vi "Get Slice Color.vi"(7 "Opacity":sgl, 9 "Normal Array":cluster{"X":sgl, "Y":sgl, "Z":sgl}[](array[cluster]), 11 "Color Pair Array":cluster{"Color":u32, "String":string}[](array[cluster])) -> (1 "Color Array":cluster{"R":sgl, "G":sgl, "B":sgl, "A":sgl}[](array[cluster]), 3 "Color Binding Mode":T1(ring))   [LabVIEW 2017, in "3D Pie.lvclass"]
uses:
  <vilib>/Math Plots/3D Math Plots/3D Pie/3D Pie/3D Pie.lvclass
  <vilib>/picture/3D Picture Control/NI_3D Picture Control.lvlib
  <vilib>/Math Plots/3D Math Plots/3D Plot/3D Plot/3D Plot.lvclass
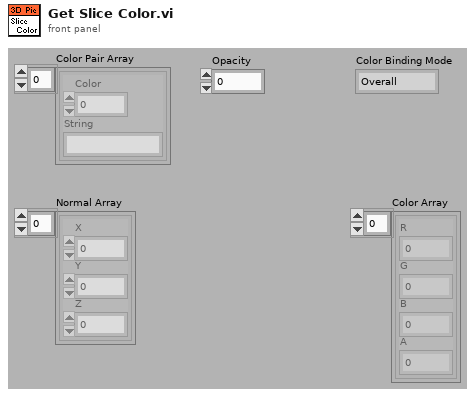
[diagram p1: front panel]
types:
  T1 = enum16{"Overall", "Per Primitive", "Per Vertex", "Binding Off"}
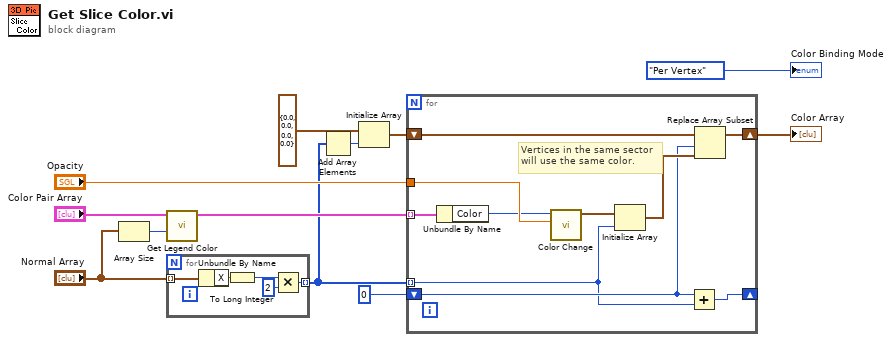
[diagram p0: block diagram]
diagram:
  n1 = Array Size(array="Normal Array") -> (size(s)=w6:i32)
  n2 = call <vilib>:"Get Legend Color.vi"("Pair Array Length"=w6, "Color Pair Array In"="Color Pair Array") -> ("Color Pair Array Out"=w8:cluster{"Color":u32, "String":string}[])  [unwired: 9 out]
  n3 = for {
    tunnel: "Normal Array" -> [w16] mode=indexing
    tunnel: [w13] -> w2 mode=indexing
    n4 = Unbundle By Name(w16) -> ("X"=w17:sgl)
    n5 = To Long Integer(number=w17) -> (32bit integer=w14:i32)
    n6 = Multiply(x=w14, y=2) -> (x*y=w13:i32)
  }
  n7 = Add Array Elements(numeric array=w2) -> (sum=w1:i32)
  n8 = Initialize Array(cluster{"R":sgl, "G":sgl, "B":sgl, "A":sgl} {"R"=0.0, "G"=0.0, "B"=0.0, "A"=0.0} ("RGBA"), w1) -> (w5:cluster{"R":sgl, "G":sgl, "B":sgl, "A":sgl}[])
  n9 = for {
    shift-right: [w26] -> w11
    shift-left: w5 -> [w27]
    tunnel: "Opacity" -> [w24]
    tunnel: w8 -> [w23] mode=indexing
    shift-right: [w19] -> _
    shift-left: 0 -> [w20]
    tunnel: w2 -> [w18] mode=indexing
    # "Vertices in the same sector\nwill use the same color."
    n10 = Unbundle By Name(w23) -> ("Color"=w22:u32)
    n11 = call <vilib>:"Color Change.vi"("Alpha"=w24, "Color"=w22) -> ("RGBA"=w25:cluster{"R":sgl, "G":sgl, "B":sgl, "A":sgl})  [unwired: 9 out]
    n12 = Initialize Array(w25, w18) -> (w21:cluster{"R":sgl, "G":sgl, "B":sgl, "A":sgl}[])
    n13 = Add(x=w20, y=w18) -> (x+y=w19:i32)
    n14 = Replace Array Subset(array=w27, new element=w21, index=w20) -> (w26:cluster{"R":sgl, "G":sgl, "B":sgl, "A":sgl}[])
  }
  "Color Array" <- w11
  "Color Binding Mode" <- T1."Per Vertex" ("Color Binding Mode")
